vi "Configure Edge Trigger Source.vi"(0 "VISA resource name":refnum<visa-resource-name>, 1 "Trigger Level (0.0)":dbl format="%^.3e", 5 "Trigger (A)":i32(ring)=1 items=["A"=1, "B"=2], 7 "Channel (Channel 1)":i32(ring)=1 items=["Channel 1"=1, "Channel 2"=2, "Channel 3"=3, "Channel 4"=4], 9 "Trigger Source (Channel 1)":i32(ring)=1 items=["Channel 1"=1, "Channel 2"=2, "Channel 3"=3, "Channel 4"=4, "External Trigger Input"=5, "AC Line"=6, "Serial Bus 1"=7, "Serial Bus 2"=8, "Serial Bus 3"=9, "Serial Bus 4"=10, "Digital 0"=11, "Digital 1"=12, "Digital 2"=13, "Digital 3"=14, "Digital 4"=15, "Digital 5"=16, "Digital 6"=17, "Digital 7"=18, "Digital 8"=19, "Digital 9"=20, "Digital 10"=21, "Digital 11"=22, "Digital 12"=23, "Digital 13"=24, "Digital 14"=25, "Digital 15"=26], 11 "error in (no error)":errorcluster, 12 "Trigger Slope (Rising Edge)":i32(ring) items=["Rising Edge", "Falling Edge", "Either"]) -> (4 "VISA resource name out":refnum<visa-resource-name>, 15 "error out":errorcluster)   [LabVIEW 2020, in "Rohde&Schwarz RTx Oscilloscopes.lvlib"]
doc: "This VI configures the trigger.\n\nAttributes:\nRSRTX_ATTR_TRIGGER_SOURCE_A\nRSRTX_ATTR_TRIGGER_SOURCE_B\nRSRTX_ATTR_TRIGGER_LEVEL_A\nRSRTX_ATTR_TRIGGER_LEVEL_B\nRSRTX_ATTR_TRIGGER_SLOPE_A\nRSRTX_ATTR_TRIGGER_SLOPE_B\n\nRemote-control commands:\nTRIGger:<Trigger>:SOURce\nTRIGger:<Trigger>:LEVel<Channel>[:VALue]\nTRIGger:{Trigger}:EDGE:SLOPe"
uses:
  Rohde&Schwarz RTx Oscilloscopes.lvlib
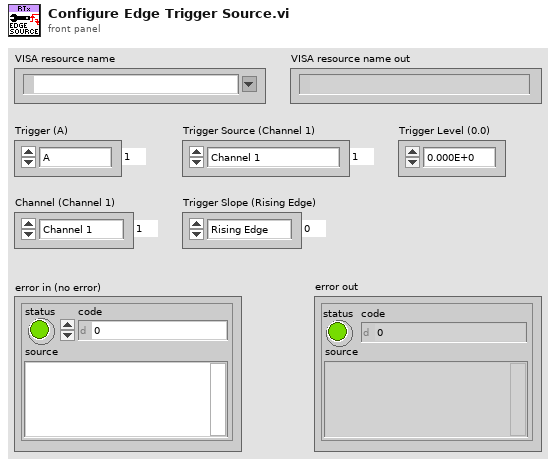
[diagram p1: front panel]
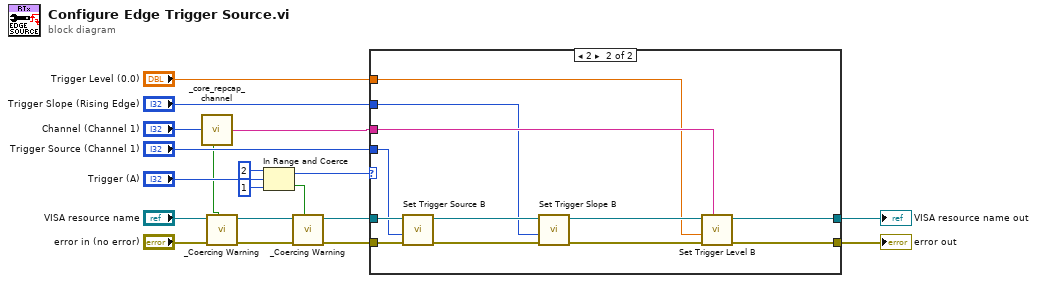
[diagram p0: block diagram]
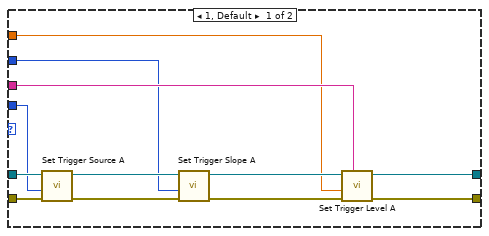
[diagram p2: hidden frame]
diagram:
  n1 = call "_core_repcap_channel.vi"("Channel In"="Channel (Channel 1)") -> ("In Range?"=w2:bool, "Channel Identifier Out"=w1:string)  [unwired: 1 out]
  n2 = call "_Coercing Warning.vi"("In Range?"=w2, "error in"="error in (no error)", "VISA resource name"="VISA resource name") -> ("error out"=w3:errorcluster, "VISA resource name out"=w5:refnum<visa-resource-name>)  [unwired: 7 in]
  n3 = In Range and Coerce(upper limit=2, x="Trigger (A)", lower limit=1) -> (coerced(x)=w8:i32, In Range?=w17:bool)
  n4 = call "_Coercing Warning.vi"("In Range?"=w17, "error in"=w3, "VISA resource name"=w5) -> ("error out"=w16:errorcluster, "VISA resource name out"=w15:refnum<visa-resource-name>)  [unwired: 7 in]
  n5 = case shown="2" w8 {
    tunnel: w16 -> [w31 w43]
    tunnel: [w27 w39] -> w9
    tunnel: [w26 w38] -> w10
    tunnel: w15 -> [w30 w42]
    tunnel: "Trigger Source (Channel 1)" -> [w20 w32]
    tunnel: "Trigger Slope (Rising Edge)" -> [w21 w33]
    tunnel: "Trigger Level (0.0)" -> [w22 w34]
    tunnel: w1 -> [w23 w35]
    frame 1, Default {
      n6 = call "Set Trigger Source A"("error in (no error)"=w31, "Trigger Source A (1 - Channel 1)"=w20, "instrument handle"=w30) -> ("error out"=w29:errorcluster, "instrument handle out"=w24:refnum<visa-resource-name>)  [unwired: 7 in]
      n7 = call "Set Trigger Slope A"("error in (no error)"=w29, "Trigger Slope A (0 - Rising Edge)"=w21, "instrument handle"=w24) -> ("error out"=w28:errorcluster, "instrument handle out"=w25:refnum<visa-resource-name>)  [unwired: 7 in]
      n8 = call "Set Trigger Level A"("Repeated Capabilities"=w23, "error in (no error)"=w28, "Trigger Level A (0.0)"=w22, "instrument handle"=w25) -> ("error out"=w27:errorcluster, "instrument handle out"=w26:refnum<visa-resource-name>)  [unwired: 6 in]
    }
    frame 2 {
      n9 = call "Set Trigger Source B"("error in (no error)"=w43, "Trigger Source B (0 - <UNDEFINED>)"=w32, "instrument handle"=w42) -> ("error out"=w41:errorcluster, "instrument handle out"=w36:refnum<visa-resource-name>)  [unwired: 7 in]
      n10 = call "Set Trigger Slope B"("error in (no error)"=w41, "Trigger Slope B (0 - Rising Edge)"=w33, "instrument handle"=w36) -> ("error out"=w40:errorcluster, "instrument handle out"=w37:refnum<visa-resource-name>)  [unwired: 7 in]
      n11 = call "Set Trigger Level B"("Repeated Capabilities"=w35, "error in (no error)"=w40, "Trigger Level B (0.0)"=w34, "instrument handle"=w37) -> ("error out"=w39:errorcluster, "instrument handle out"=w38:refnum<visa-resource-name>)  [unwired: 6 in]
    }
  }
  "error out" <- w9
  "VISA resource name out" <- w10
